vi "global variable.vi"() -> ()   [LabVIEW 2015]
panel:
  out "Variable1":string
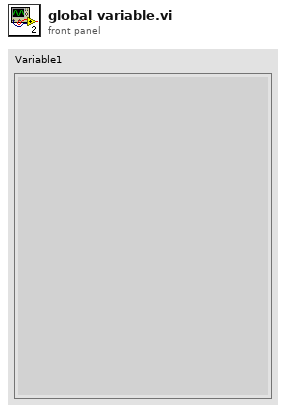
[diagram p1: front panel]
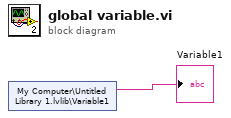
[diagram p0: block diagram]
diagram:
  n1 = shared-variable "My Computer\\Untitled Library 1.lvlib\\Variable1"() -> (→"Variable1":string)  [unwired: 1 in, 1 out]
